vi "Get JSON Data.vi"(6 "Force Hide":bool, 7 "Evaluate Pane Move":bool, 8 "error in (no error)":errorcluster, 9 "Force Get All Data":bool, 10 "VI Reference":refnum<vi>, 11 "Graph In":refnum<class "Graph.lvclass">) -> (0 "error out":errorcluster, 2 "JSON string":string, 3 "Graph Out":refnum<class "Graph.lvclass">)   [LabVIEW 2017, in "Front Panel Publisher.lvlib" / "Graph.lvclass"]
uses:
  Graph.lvclass
  Object_class/Object.lvclass
  Control_class/Control.lvclass
  Web Front Panel_class/Controls/Enum - Control Display Mode.ctl
  Web Front Panel_class/Web Front Panel.lvclass
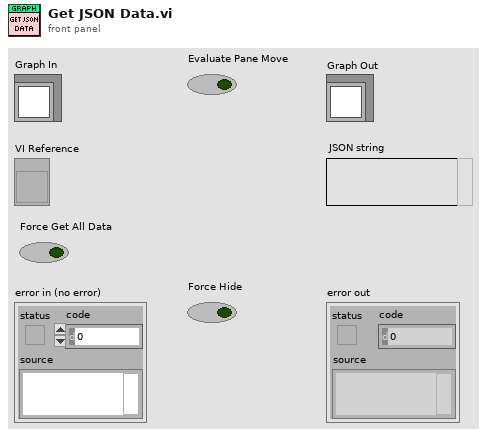
[diagram p1: front panel]
types:
  T1 = typedef "Front Panel Publisher.lvlib/Web Front Panel.lvclass/Enum - Control Display Mode.ctl" = enum16{"Value Only", "Value and Visibility", "Boolean Value Only", "Boolean Value and Visibility", "Control is Image", "Image and Visibility"}
  T2 = typedef "Front Panel Publisher.lvlib/Object.lvclass/Attributes.ctl" = cluster{"UID":i32, "Type":string, "Starting Location":T3, "Reference":refnum<vi>, "Cluster Component":bool, "Starting Rect Position":cluster{"Left":i16, "Top":i16}, "Owning Pane":refnum<vi>, "Master Total Rect Delta":T4}
  T3 = typedef "Front Panel Publisher.lvlib/Object.lvclass/Coordinates.ctl" = cluster{"Left":i32, "Top":i32, "Height":u32, "Width":u32}
  T4 = typedef "LVRectTypeDef.ctl" = cluster{"Left":i16, "Top":i16, "Right":i16, "Bottom":i16}
  T5 = typedef "Front Panel Publisher.lvlib/Control.lvclass/Attributes.ctl" = cluster{"Description":string, "Indicator":bool, "Default Value":variant, "Control Index":i32, "Label":refnum<class "Text.lvclass">, "Caption":refnum<class "Text.lvclass">, "Image b64":string, "No Control Index":bool, "Display Mode":T1}
  T6 = typedef "Front Panel Publisher.lvlib/Graph.lvclass/Attributes.ctl" = cluster{"X Label Text":string, "X Format String":string, "Y Label Text":string[], "Y Format String":string[], "Plot Y Axis Selection":enum16{"Y Axis", "Y2 Axis"}[], "Width":u32, "Series JSON Data":string}
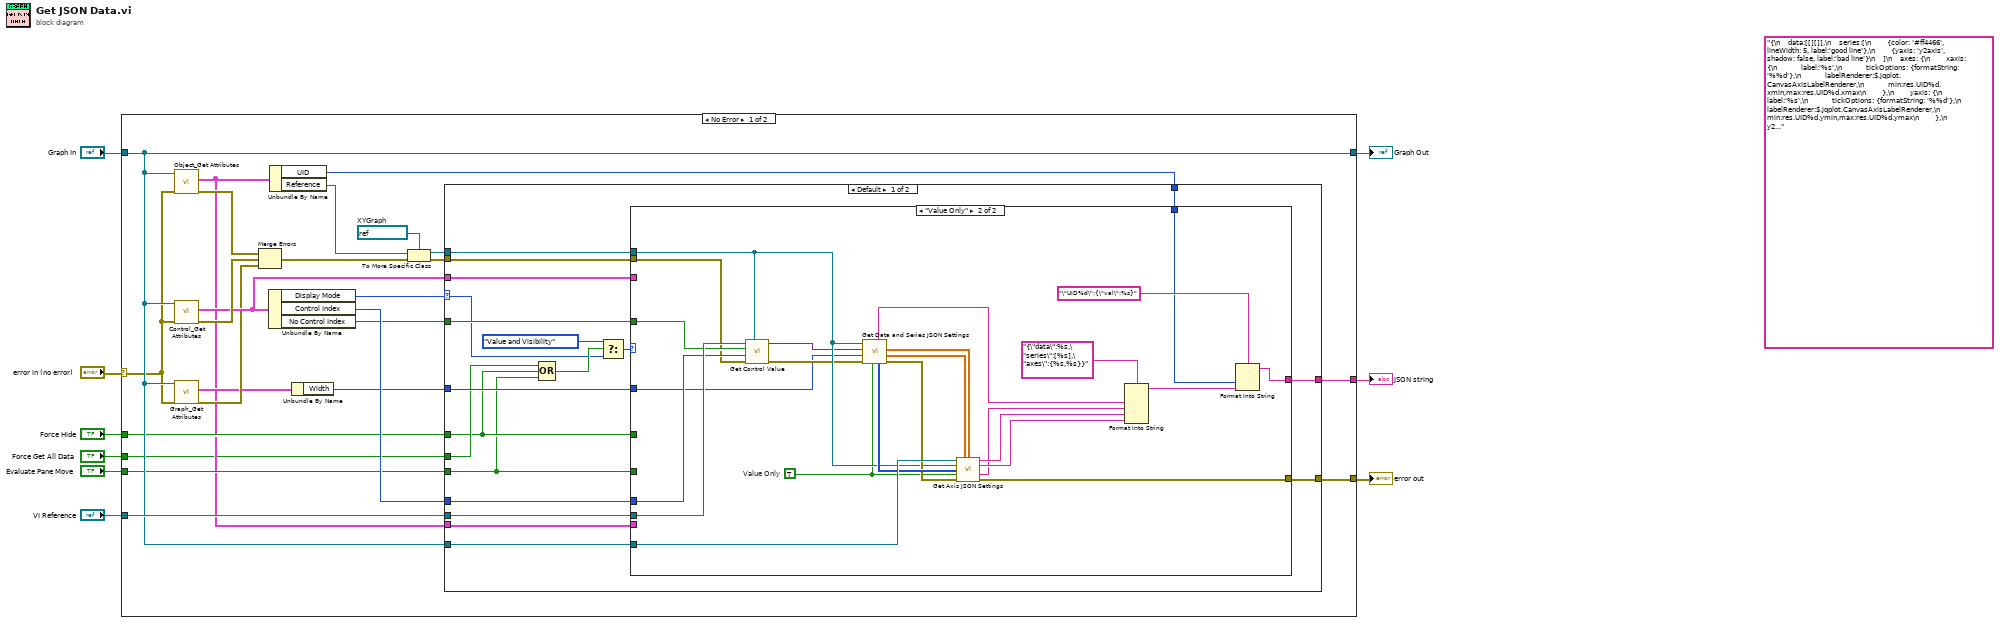
[diagram p0: block diagram]
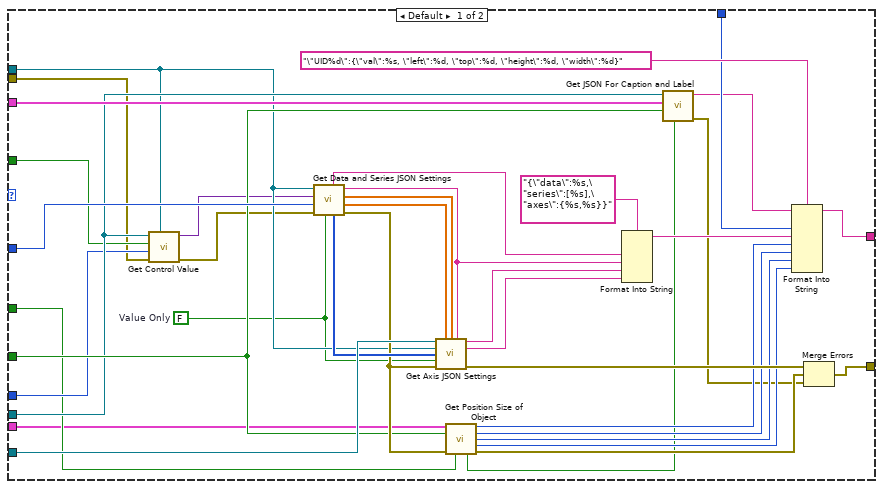
[diagram p2: hidden frame]
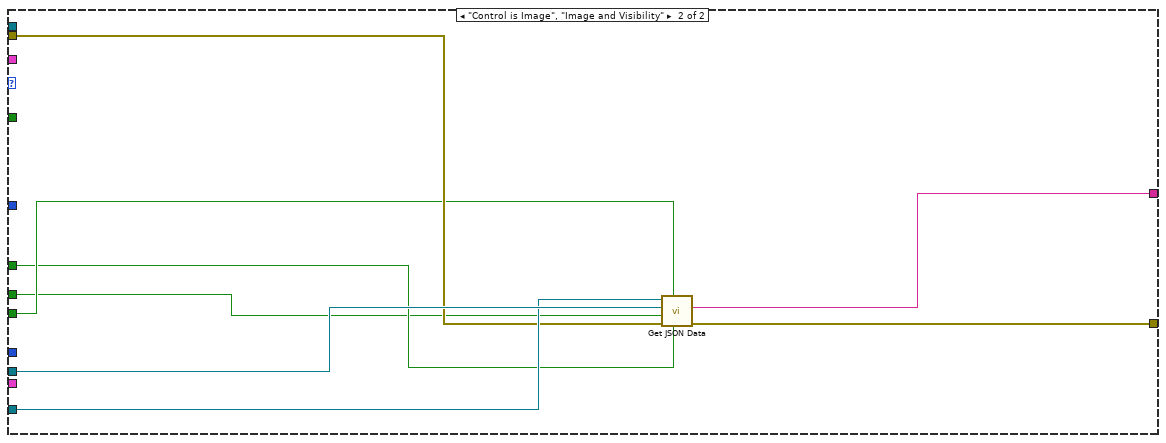
[diagram p3: hidden frame]
diagram:
  (unwired) "{\n    data:[[][]],\n    series:[\n        {color: '#ff4466', lineWidth: 5, label:'good line'},\n        {yaxis: 'y2axis', shadow: false, label:'bad line'}\n    ]\n    axes: {\n        xaxis: {\n            label:'%s',\n            tickOptions: {formatString: '%%d'},\n            labelRenderer:$.jqplot.CanvasAxisLabelRenderer,\n            min:res.UID%d.xmin,max:res.UID%d.xmax\n        },\n        yaxis: {\n            label:'%s',\n            tickOptions: {formatString: '%%d'},\n            labelRenderer:$.jqplot.CanvasAxisLabelRenderer,\n            min:res.UID%d.ymin,max:res.UID%d.ymax\n        },\n        y2axis: {\n            label:'%s',\n            tickOptions: {formatString: '%%d'},\n            labelRenderer:$.jqplot.CanvasAxisLabelRenderer\n        }\n      resetAxes:true\n    }\n}"
  n1 = case shown="No Error" "error in (no error)" {
    selector: "error in (no error)" -> [w18 w123]
    tunnel: [w23 w123] -> w8
    tunnel: [w19 w122] -> w6
    tunnel: "Graph In" -> [w19 w122]
    tunnel: [w21 _] -> w5
    tunnel: "Force Get All Data" -> [w10 _]
    tunnel: "VI Reference" -> [w24 _]
    tunnel: "Evaluate Pane Move" -> [w14 _]
    tunnel: "Force Hide" -> [w12 _]
    frame No Error {
      w32 = refnum<vi> refnum  # XYGraph
      n2 = call "Object_Get Attributes.vi"("error in (no error)"=w18, "Object In"=w19) -> ("error out"=w29:errorcluster, "Object Attributes"=w11:T2)  [unwired: 7 in, 1 out]
      n3 = call "Control_Get Attributes.vi"("error in (no error)"=w18, "Control In"=w19) -> ("error out"=w30:errorcluster, "Control Attributes"=w20:T5)  [unwired: 7 in, 1 out]
      n4 = call "Graph_Get Attributes.vi"("error in (no error)"=w18, "reference in"=w19) -> ("error out"=w17:errorcluster, "Graph Attributes"=w16:T6)  [unwired: 6 in, 2 out]
      n5 = Merge Errors(w29, w30, w17) -> (w28:errorcluster)
      n6 = Unbundle By Name(w20) -> ("Display Mode"=w27:T1, "Control Index"=w25:i32, "No Control Index"=w13:bool)
      n7 = Unbundle By Name(w11) -> ("UID"=w22:i32, "Reference"=w26:refnum<vi>)
      n8 = Unbundle By Name(w16) -> ("Width"=w15:u32)
      n9 = To More Specific Class(target class=w32, reference=w26, error in=w28) -> (specific class reference=w31:refnum<vi>, error out=w33:errorcluster)
      n10 = case shown="Default" w27 {
        selector: w27 -> [w38 _]
        tunnel: [w52 w119] -> w23
        tunnel: w33 -> [w51 w118]
        tunnel: w31 -> [w50 _]
        tunnel: [w49 w117] -> w21
        tunnel: w19 -> [w48 w120]
        tunnel: w25 -> [w47 _]
        tunnel: w24 -> [w46 w121]
        tunnel: w22 -> [w45 _]
        tunnel: w20 -> [w44 _]
        tunnel: w15 -> [w43 _]
        tunnel: w14 -> [w35 w116]
        tunnel: w13 -> [w42 _]
        tunnel: w12 -> [w36 w115]
        tunnel: w11 -> [w41 _]
        tunnel: w10 -> [w37 w114]
        frame Default {
          n11 = Compound Arithmetic op=OR(w37, w36, w35) -> (w39:bool)
          n12 = Select(t=Enum_-_Control_Display_Mode."Value and Visibility", s=w39, f=w38) -> (s? t:f=w34:T1)
          n13 = case shown="\"Value Only\"" w34 {
            tunnel: [w77 w105] -> w52
            tunnel: w51 -> [w60 w95]
            tunnel: w50 -> [w61 w97]
            tunnel: [w70 w101] -> w49
            tunnel: w48 -> [w85 w110]
            tunnel: w47 -> [w63 w98]
            tunnel: w46 -> [w64 w99]
            tunnel: w45 -> [w79 w103]
            tunnel: w44 -> [w68 _]
            tunnel: w43 -> [w67 w92]
            tunnel: w35 -> [w65 _]
            tunnel: w42 -> [w62 w96]
            tunnel: w36 -> [w57 _]
            tunnel: w41 -> [w56 _]
            frame Default {
              w53 = FALSE  # Value Only
              n14 = call "Get Control Value.vi"("Control Reference"=w61, "error in (no error)"=w60, "Control Index"=w63, "No Control Index"=w62, "VI Reference"=w64) -> ("error out"=w59:errorcluster, "Variant"=w58:variant)  [unwired: 5 in]
              n15 = call "Get Data and Series JSON Settings.vi"("Value Only"=w53, "error in (no error)"=w59, "Width"=w67, "XY Data"=w58, "XYGraph in"=w61) -> ("error out"=w78:errorcluster, "Minimums"=w82:dbl[], "Maximums"=w83:dbl[], "Series JSON"=w66:string, "Plot Y Scale Index"=w84:u32[], "Data JSON"=w86:string)  [unwired: 1 in]
              n16 = call "Get Axis JSON Settings.vi"("Graph In"=w85, "Minimums"=w82, "Maximums"=w83, "Series JSON In"=w66, "XYGraph Refnum"=w61, "Plot Y Scale Index"=w84, "Value Only"=w53, "error in (no error)"=w78) -> ("X Axis Settings"=w89:string, "Y Axis Settings"=w88:string, "error out"=w81:errorcluster)  [unwired: 4 in, 1 out]
              n17 = call "Get Position Size of Object.vi"("Object Attributes"=w56, "Evaluate Pane Move"=w65, "error in (no error)"=w78, "Force Hide"=w57) -> ("Left"=w75:i32, "Top"=w74:i32, "Height"=w73:u32, "Width"=w72:u32, "Hidden"=w55:bool, "error out"=w76:errorcluster)  [unwired: 6 in]
              n18 = Format Into String(format string="{\"data\":%s,\"series\":[%s],\"axes\":{%s,%s}}", w86, w66, w89, w88) -> (resulting string=w71:string)  [unwired: 2 in, 1 out]
              n19 = call "Get JSON For Caption and Label.vi"("Force Hide"=w55, "Evaluate Pane Move"=w65, "Data"=w68, "VI in"=w64) -> ("error out"=w54:errorcluster, "JSON"=w69:string)  [unwired: 6 in]
              n20 = Format Into String(format string="\"UID%d\":{\"val\":%s, \"left\":%d, \"top\":%d, \"height\":%d, \"width\":%d}", initial string=w69, w79, w71, w75, w74, w73, w72) -> (resulting string=w70:string)  [unwired: 1 in, 1 out]
              n21 = Merge Errors(w81, w76, w54) -> (w77:errorcluster)
            }
            frame "Value Only" {
              w91 = TRUE  # Value Only
              n22 = call "Get Control Value.vi"("Control Reference"=w97, "error in (no error)"=w95, "Control Index"=w98, "No Control Index"=w96, "VI Reference"=w99) -> ("error out"=w94:errorcluster, "Variant"=w93:variant)  [unwired: 5 in]
              n23 = call "Get Data and Series JSON Settings.vi"("Value Only"=w91, "error in (no error)"=w94, "Width"=w92, "XY Data"=w93, "XYGraph in"=w97) -> ("error out"=w106:errorcluster, "Minimums"=w107:dbl[], "Maximums"=w108:dbl[], "Plot Y Scale Index"=w109:u32[], "Data JSON"=w90:string)  [unwired: 1 in, 1 out]
              n24 = call "Get Axis JSON Settings.vi"("Graph In"=w110, "Minimums"=w107, "Maximums"=w108, "XYGraph Refnum"=w97, "Plot Y Scale Index"=w109, "Value Only"=w91, "error in (no error)"=w106) -> ("X Axis Settings"=w113:string, "Y Axis Settings"=w112:string, "Series JSON Out"=w100:string, "error out"=w105:errorcluster)  [unwired: 5 in]
              n25 = Format Into String(format string="{\"data\":%s,\"series\":[%s],\"axes\":{%s,%s}}", w90, w100, w113, w112) -> (resulting string=w102:string)  [unwired: 2 in, 1 out]
              n26 = Format Into String(format string="\"UID%d\":{\"val\":%s}", w103, w102) -> (resulting string=w101:string)  [unwired: 2 in, 1 out]
            }
          }
        }
        frame "Control is Image", "Image and Visibility" {
          n27 = call-parent "Get JSON Data.vi"("Force Hide"=w115, "Evaluate Pane Move"=w116, "error in (no error)"=w118, "Force Get All Data"=w114, "VI Reference"=w121, "Control In"=w120) -> ("error out"=w119:errorcluster, "JSON string"=w117:string)  [unwired: 3 in, 1 out]
        }
      }
    }
    frame Error {
    }
  }
  "error out" <- w8
  "Graph Out" <- w6
  "JSON string" <- w5
